vi "AssertOnlyFalse-Issue92.vi"(8 "error in":errorcluster) -> (0 "error out":errorcluster)   [LabVIEW 2013]
uses:
  classes/Assert/Assert Not Error.vi
  classes/Test/Test.lvclass
  classes/Assert/Assert.lvclass
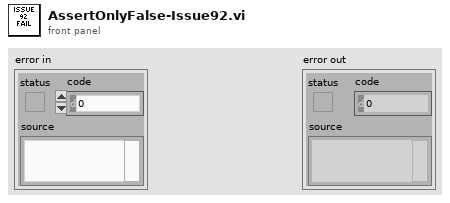
[diagram p1: front panel]
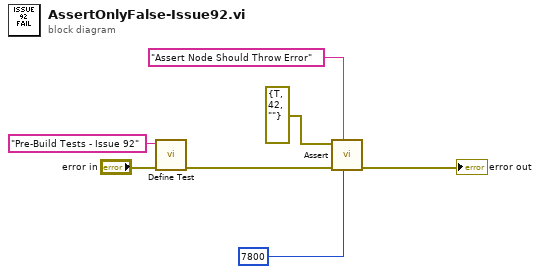
[diagram p0: block diagram]
diagram:
  n1 = call "Define Test.vi"("error in (no error)"="error in", "Label (VI Title)"="Pre-Build Tests - Issue 92") -> ("error out"=w6:errorcluster)  [unwired: 9 in]
  n2 = call-poly "Assert.vi"("error code (1)"=7800, "Label"="Assert Node Should Throw Error", "error in (no error)"=w6, "Not Error?"=errorcluster {"status"=TRUE, "code"=42, "source"=""}) -> ("error out"=→"error out":errorcluster)  [unwired: 7 in]
